vi "Photon-STR18_2_1.vi"() -> ()   [LabVIEW 2015]
uses:
  subVi/Menu.ctl
  <vilib>/Utility/file.llb/Write Delimited Spreadsheet (DBL).vi
panel:
  out "Size B":dbl
  out "Size A":dbl
  out "Duration A":dbl format="%.4f"
  out "Duration B":dbl format="%.4f"
  out "Total # of photons B":dbl
  out "Total # of photons A":dbl
  in  "Sample Time":i32=2
  out "b AxB":dbl format="%.4f"
  out "Correlacion 2":cluster{ext[], ext[]}(graph)
  out "< B >":dbl format="%.4f"
  out "< A >":dbl format="%.4f"
  out "Structura corregida":cluster{ext[], ext[]}(graph)
  in  "P":i32=64
  out "Numeric":i32
  out "sum A":dbl format="%#_10g"
  out "sum B":dbl format="%#_10g"
  out "Correlacion":cluster{ext[], ext[]}(graph)
  out "# of Channels":i32
  out "Duration":sgl
  in  "m":i32=2
  out "time":ext[](array[numeric])
  out "corr":ext[](array[numeric])
  out "d*(k)":dbl[][](array[numeric])
  out "Structura":cluster{ext[], ext[]}(graph)
  out "g(k) lineal":ext[](array[numeric])
  out "millisecond timer value":u32
  in  "EXIT":bool
  in  "Open File":bool
  in  "Analysis":u16(ring) items=["Auto correlation", "Cross correlation AxB"]
  out "elapsed time in min":dbl
  out "Elapsed time (s)":dbl
  # "PhotonSTR-18"
  # "Parameters"
  # "Output"
  # "Channel A"
  # "Channel B"
  # "V2.1"
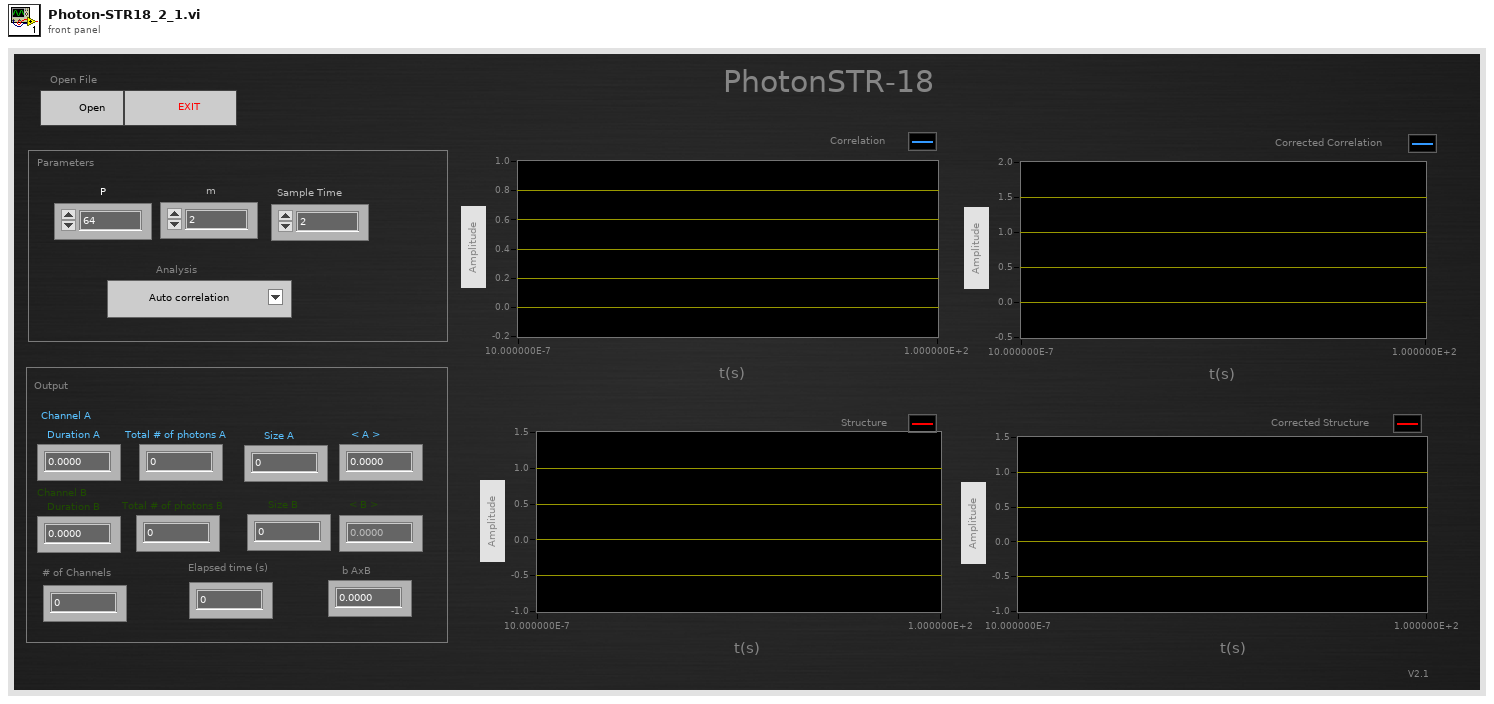
[diagram p1: front panel]
types:
  T1 = typedef "Menu.ctl" = enum16{"Init", "user action", "Load file", "Select range", "Process Photons(t)", "Process Segmentation", "Process Correlation ", "Save data", "Stop"}
  T2 = enum16{"open", "replace", "create", "open or create", "replace or create", "replace or create with confirmation"}
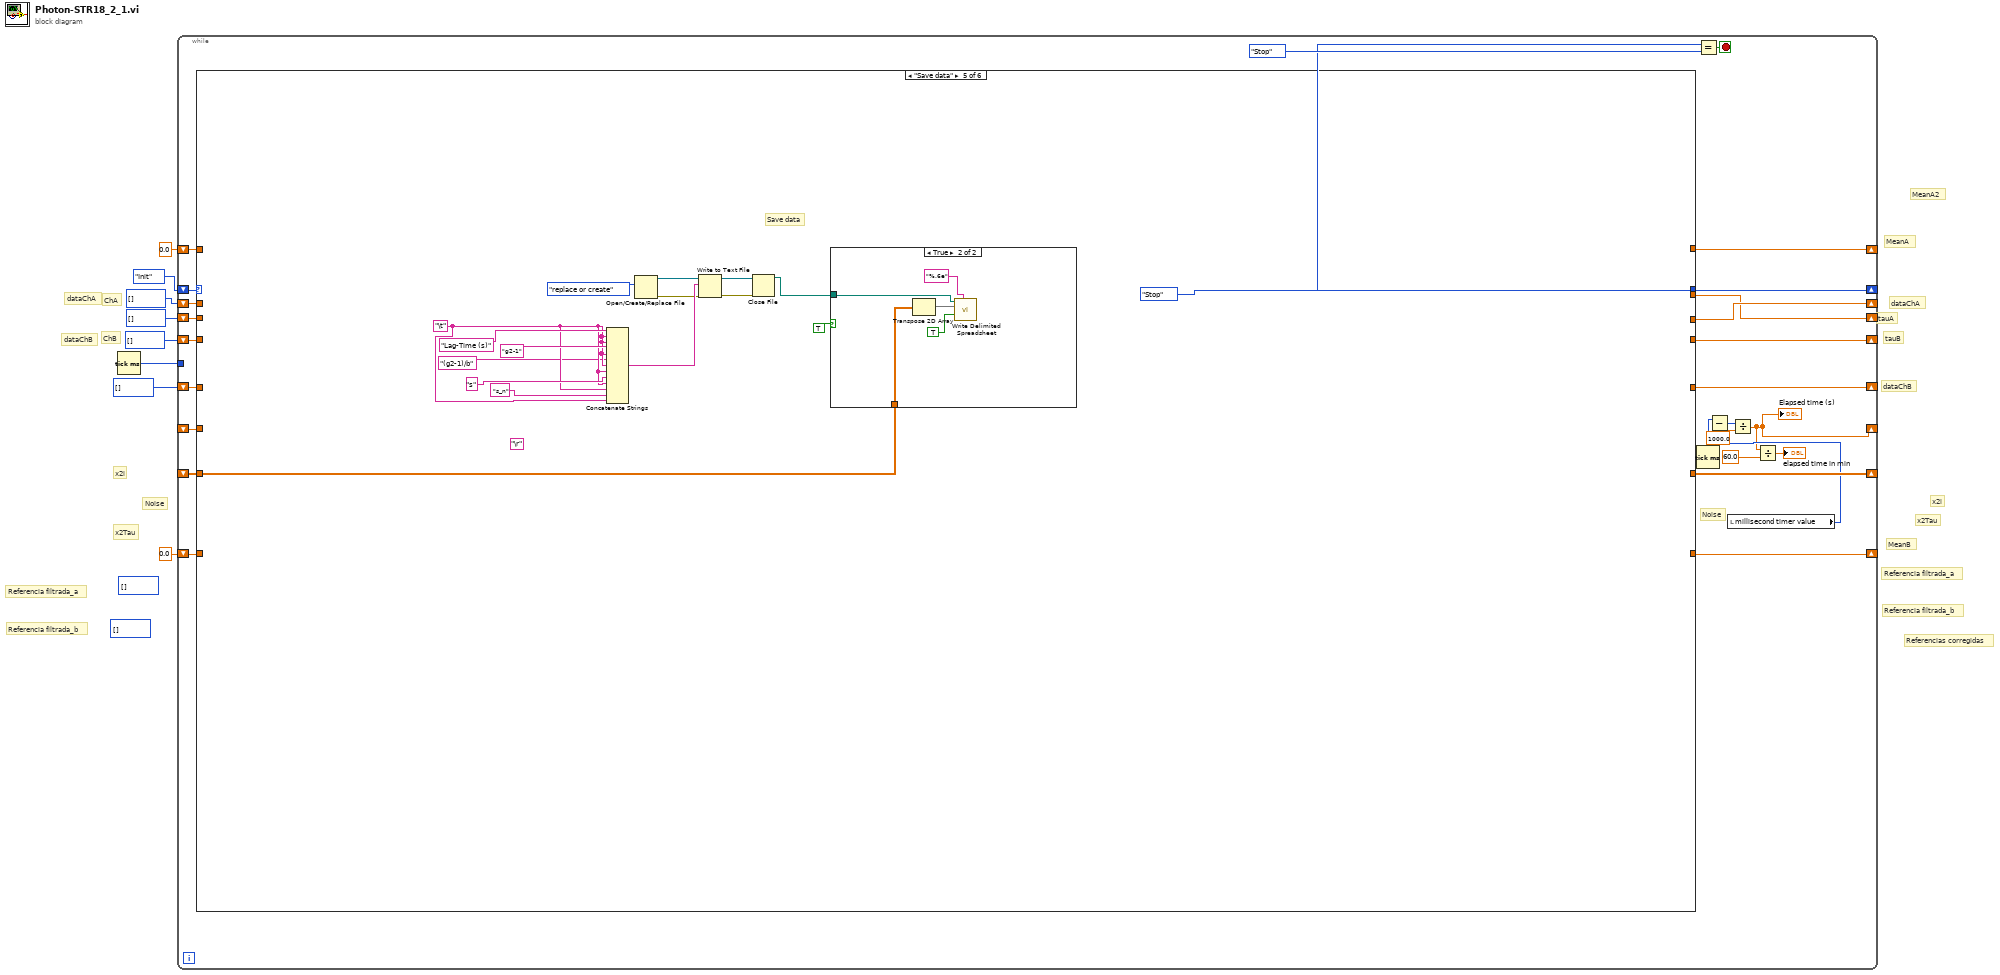
[diagram p0: block diagram]
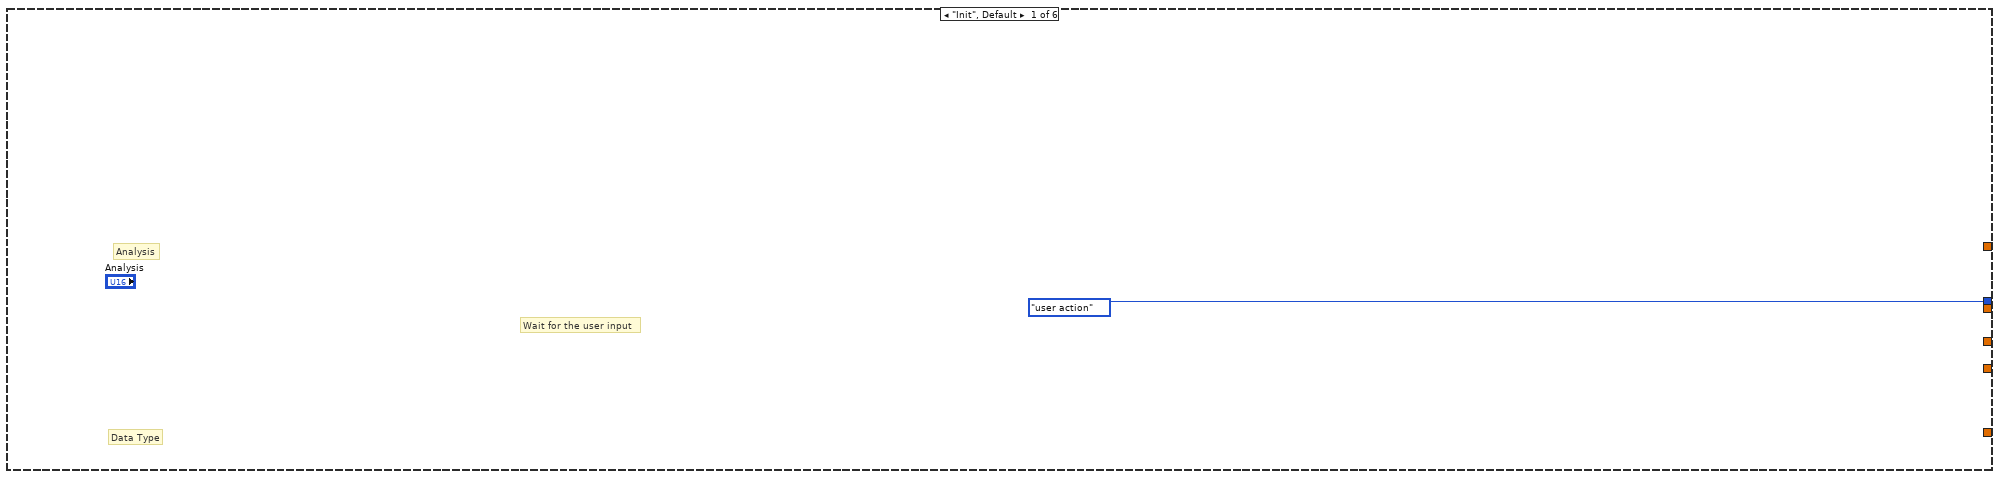
[diagram p2: hidden frame]
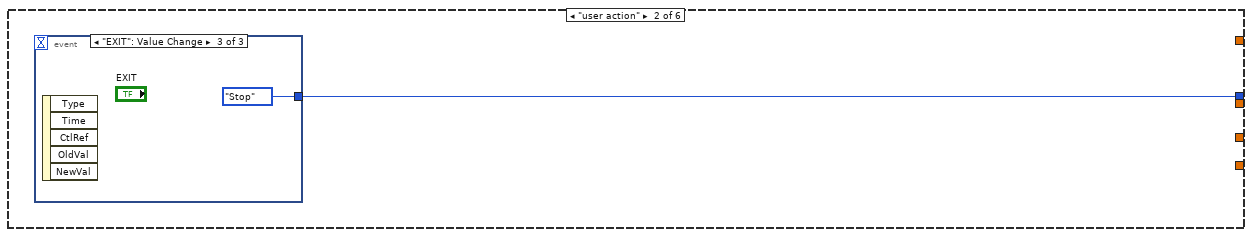
[diagram p3: hidden frame]
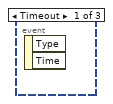
[diagram p4: hidden frame]
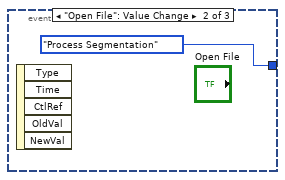
[diagram p5: hidden frame]
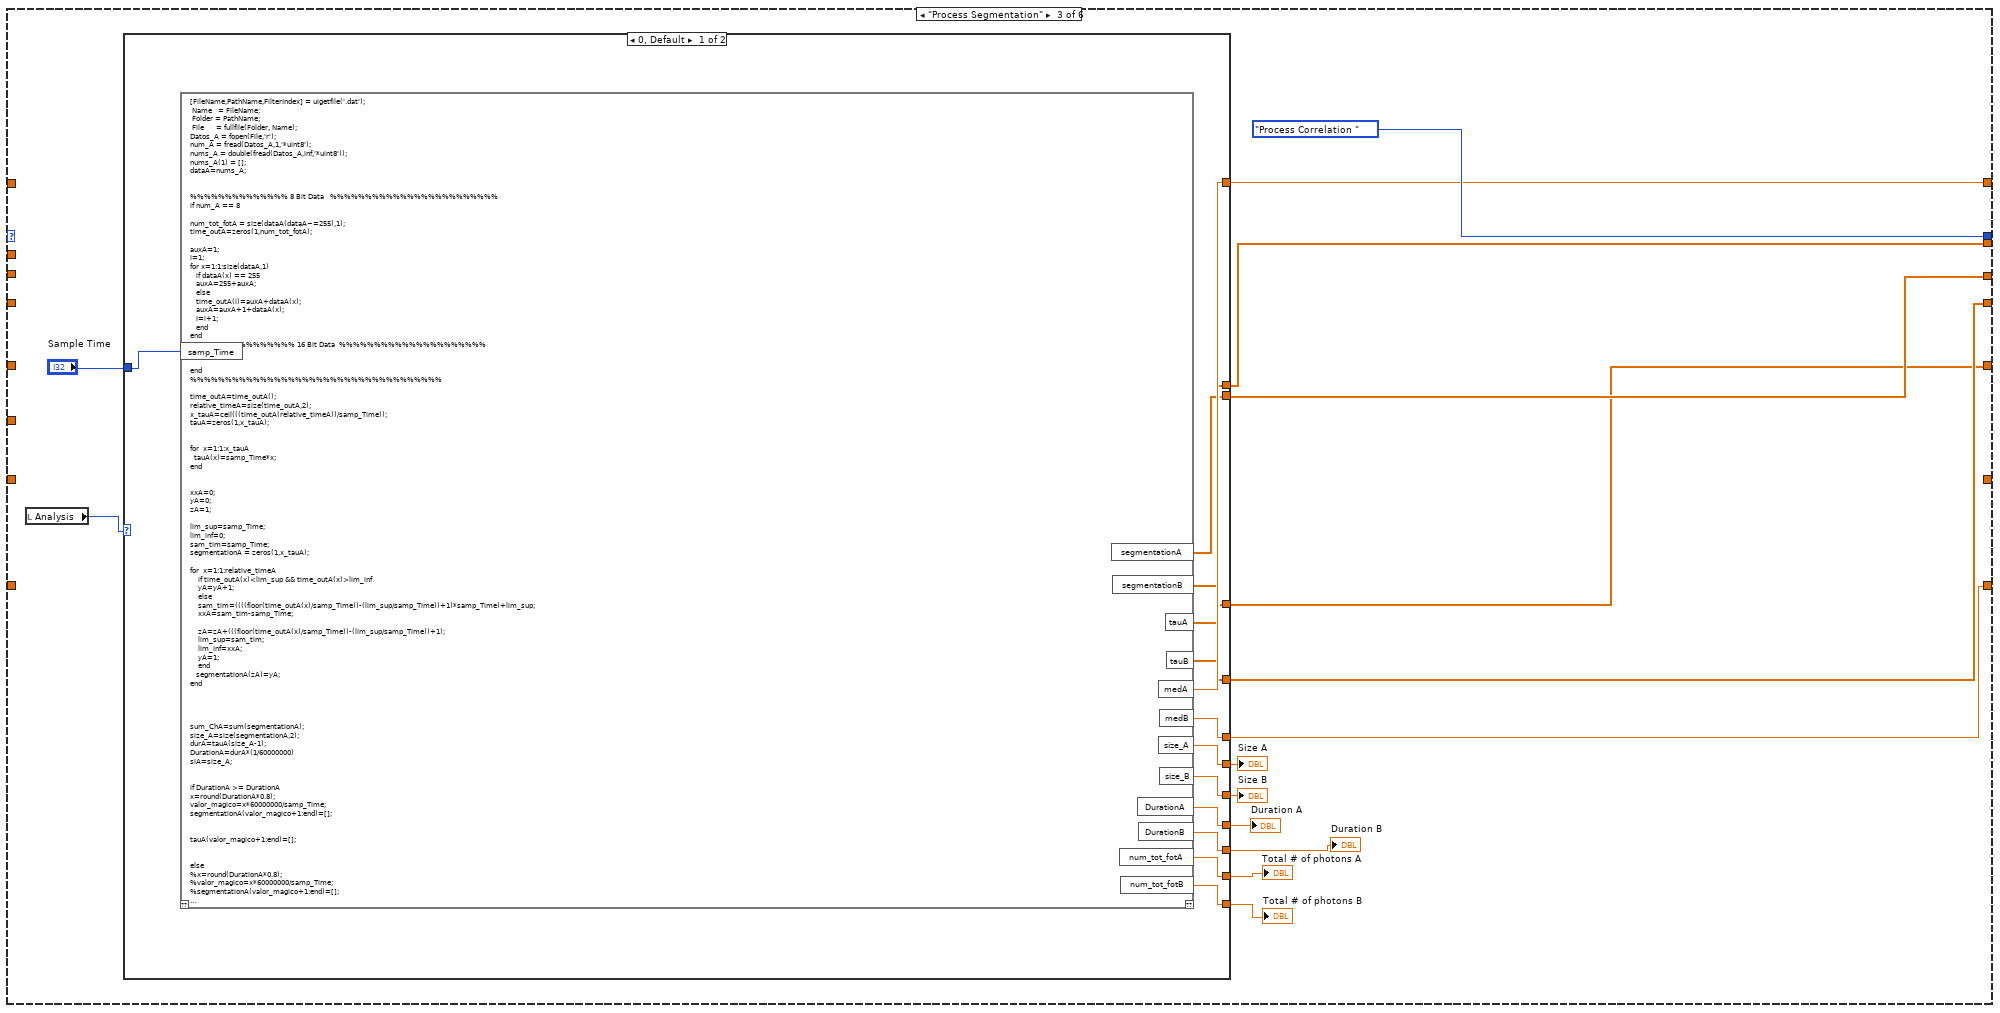
[diagram p6: hidden frame]
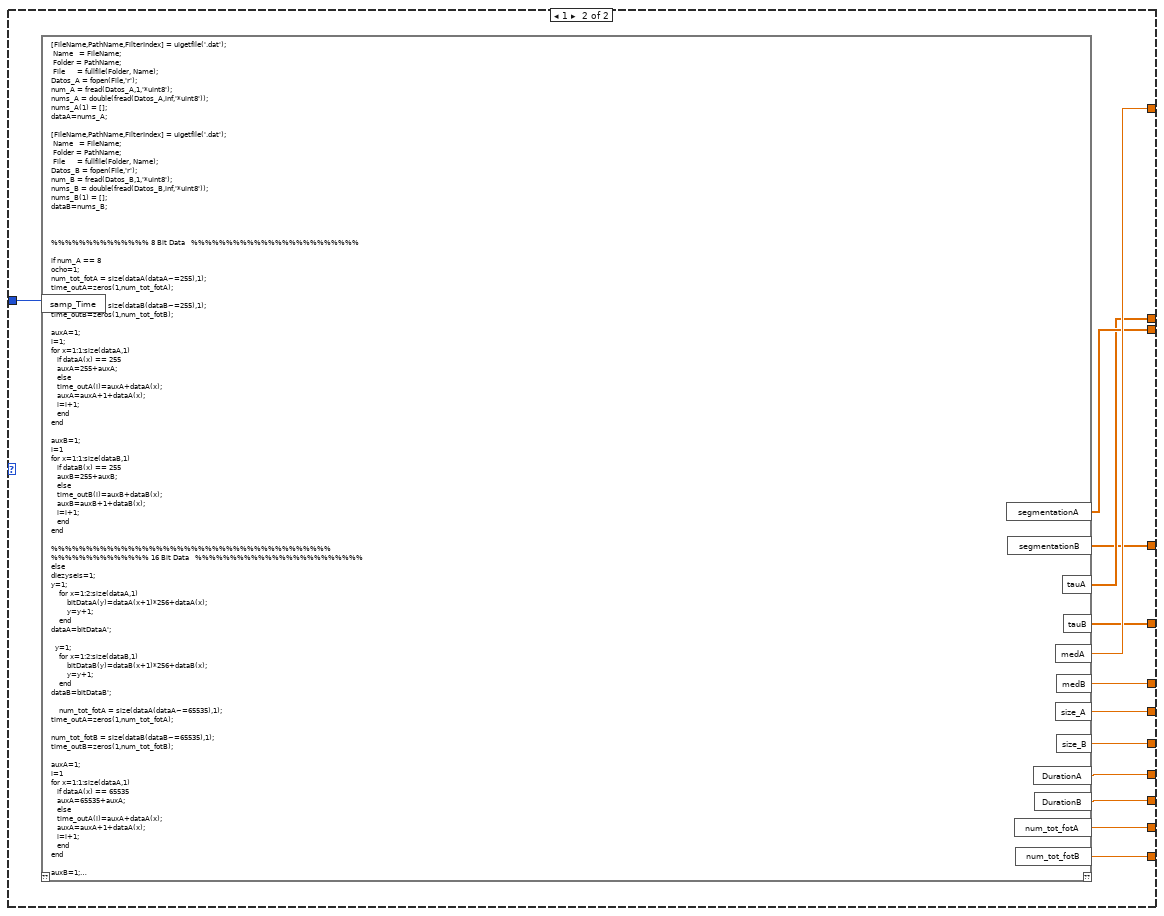
[diagram p7: hidden frame]
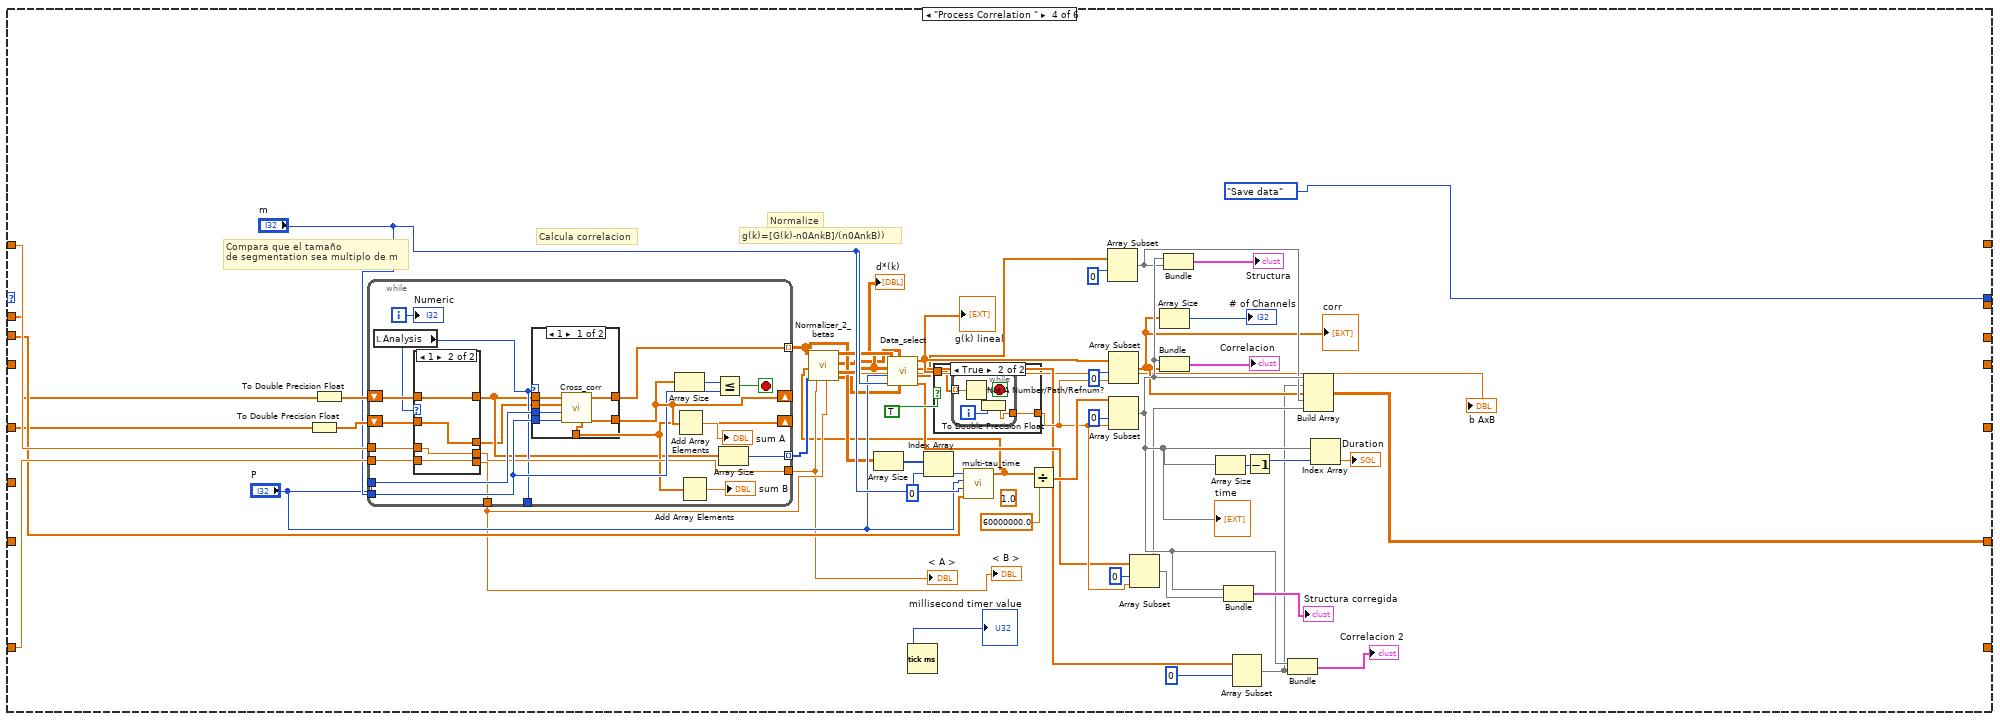
[diagram p8: hidden frame]
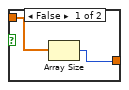
[diagram p9: hidden frame]
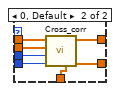
[diagram p10: hidden frame]
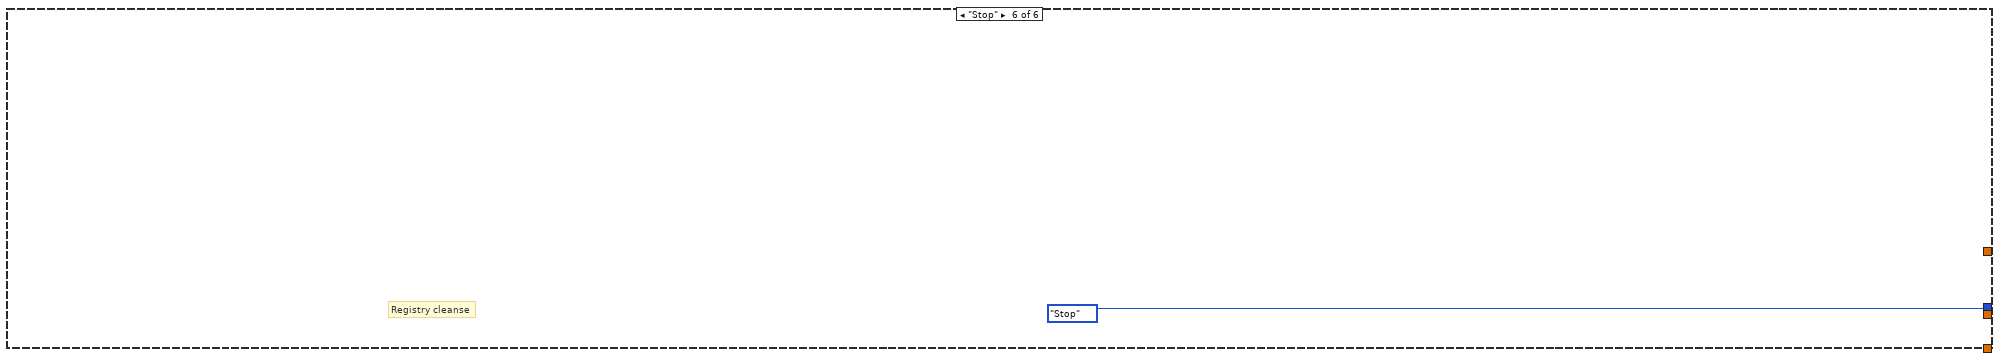
[diagram p13: hidden frame]
diagram:
  (unwired) u32[] [] ("Photon trace A")
  (unwired) u32[] [] ("Photon trace A")
  # "dataChB"
  # "dataChA"
  # "Referencias corregidas"
  # "Referencia filtrada_b"
  # "Referencia filtrada_a"
  # "Referencia filtrada_b"
  # "Referencia filtrada_a"
  # "Noise"
  # "x2Tau"
  # "x2i"
  # "x2Tau"
  # "x2i"
  # "MeanA2"
  # "MeanB"
  # "MeanA"
  # "tauB"
  # "tauA"
  # "ChB"
  # "dataChB"
  # "dataChA"
  # "ChA"
  n1 = Tick Count (ms)() -> (millisecond timer value=w5:u32)
  n2 = while {
    shift-right: [w32] -> _
    shift-left: Menu."Init" ("Menu") -> [w34]
    shift-right: [w30] -> _
    shift-left: u32[] [] ("Photon trace A") -> [w29]
    shift-right: [w28] -> _
    shift-left: u32[] [] ("Photon trace A") -> [w27]
    shift-right: [w16] -> _
    shift-left: _ -> [w26]
    tunnel: w5 -> [_]
    shift-right: [w20] -> _
    shift-left: u32[] [] ("Photon trace A") -> [w19]
    shift-right: [w18] -> _
    shift-left: u32[] [] ("Photon trace A") -> [w17]
    shift-right: [w13] -> _
    shift-left: _ -> [w15]
    shift-right: [w12] -> _
    shift-left: 0.0 ("mean") -> [w10]
    shift-right: [w11] -> _
    shift-left: 0.0 ("mean") -> [w9]
    stop <- w31 stop-if-true
    # "Noise"
    n3 = case shown="\"Save data\"" w34 {
      tunnel: [Menu."user action" ("Menu") w36 Menu."Process Correlation " ("Menu") Menu."Save data" ("Menu") Menu."Stop" ("Menu") Menu."Stop" ("Menu")] -> w32
      tunnel: [_ _ w42 _ _ _] -> w30
      tunnel: w29 -> [_ _ _ w83 _ _]
      tunnel: [_ _ w39 _ _ _] -> w28
      tunnel: w27 -> [_ _ _ w109 _ _]
      tunnel: [_ _ _ w129 _ _] -> w16
      tunnel: w26 -> [_ _ _ _ w195 _]
      tunnel: [_ _ w41 _ _ _] -> w20
      tunnel: w19 -> [_ _ _ _ _ _]
      tunnel: [_ _ w40 _ _ _] -> w18
      tunnel: w17 -> [_ _ _ w105 _ _]
      tunnel: w15 -> [_ _ _ _ _ _]
      tunnel: [_ _ w51 _ _ _] -> w12
      tunnel: [_ _ w50 _ _ _] -> w11
      tunnel: w10 -> [_ _ _ w128 _ _]
      tunnel: w9 -> [_ _ _ w127 _ _]
      frame "Init", Default {
        # "Data Type"
        # "Analysis"
        # "Wait for the user input"
      }
      frame "user action" {
        n4 = event shown="[2] \"EXIT\": Value Change" {
          selector: _ -> [_ _ _]
          dyn-events: _ -> [_ _ _]
          timeout: _ -> [_ _ _]
          tunnel: [_ Menu."Process Segmentation" ("Menu") Menu."Stop" ("Menu")] -> w36
          event Timeout {
            n5 = event-data() -> ()  [unwired: 1 in, 2 out]
          }
          event "Open File": Value Change {
            n6 = event-data() -> ()  [unwired: 1 in, 5 out]
          }
          event "EXIT": Value Change {
            n7 = event-data() -> ()  [unwired: 1 in, 5 out]
          }
        }
      }
      frame "Process Segmentation" {
        n8 = local read "Analysis"() -> (w43:u16)
        n9 = case shown="0, Default" w43 {
          tunnel: "Sample Time" -> [w66 w79]
          tunnel: [w58 w78] -> w51
          tunnel: [w59 w77] -> w50
          tunnel: [w64 w76] -> w49
          tunnel: [w65 w75] -> w48
          tunnel: [w61 w74] -> w47
          tunnel: [w60 w73] -> w46
          tunnel: [w56 w72] -> w42
          tunnel: [w57 w71] -> w39
          tunnel: [w54 w70] -> w41
          tunnel: [w55 w69] -> w40
          tunnel: [w62 w68] -> w45
          tunnel: [w63 w67] -> w44
          frame 0, Default {
            n10 = script code="[FileName,PathName,FilterIndex] = uigetfile('.dat');\n Name   = FileName;\n Folder = PathName;\n File      = fullfile(Folder, Name);         \nDatos_A = fopen(File,'r');  \nnum_A = fread(Datos_A,1,'*uint8');\nnums_A = double(fread(Datos_A,inf,'*uint8'));\nnums_A(1) = []; \ndataA=nums_A;\n\n\n%%%%%%%%%%%%%% 8 Bit Data   %%%%%%%%%%%%%%%%%%%%%%%%\nif num_A == 8 \n\nnum_tot_fotA = size(dataA(dataA~=255),1); \ntime_outA=zeros(1,num_tot_fotA);\n\nauxA=1;\ni=1;\nfor x=1:1:size(dataA,1)\n   if dataA(x) == 255\n   auxA=255+auxA;    \n   else\n   time_outA(i)=auxA+dataA(x);\n   auxA=auxA+1+dataA(x);   \n   i=i+1;\n   end\nend\n%%%%%%%%%%%%%%% 16 Bit Data  %%%%%%%%%%%%%%%%%%%%%\n\n\nend\n%%%%%%%%%%%%%%%%%%%%%%%%%%%%%%%%%%%%\n\ntime_outA=time_outA();\nrelative_timeA=size(time_outA,2);\nx_tauA=ceil(((time_outA(relative_timeA))/samp_Time));\ntauA=zeros(1,x_tauA);\n\n\nfor  x=1:1:x_tauA\n  tauA(x)=samp_Time*x;   \nend\n\n\nxxA=0;\nyA=0;\nzA=1;\n\nlim_sup=samp_Time;\nlim_inf=0;\nsam_tim=samp_Time;\nsegmentationA = zeros(1,x_tauA);\n\nfor  x=1:1:relative_timeA\n    if time_outA(x)<lim_sup && time_outA(x)>lim_inf\n    yA=yA+1;    \n    else\n    sam_tim=((((floor(time_outA(x)/samp_Time))-(lim_sup/samp_Time))+1)*samp_Time)+lim_sup;\n    xxA=sam_tim-samp_Time;\n    \n    zA=zA+(((floor(time_outA(x)/samp_Time))-(lim_sup/samp_Time))+1);\n    lim_sup=sam_tim;\n    lim_inf=xxA;    \n    yA=1;\n    end    \n   segmentationA(zA)=yA;\nend \n                          \n\n\n\nsum_ChA=sum(segmentationA);\nsize_A=size(segmentationA,2);\ndurA=tauA(size_A-1);\nDurationA=durA*(1/60000000)\nsiA=size_A;\n\n\nif DurationA >= DurationA\nx=round(DurationA*0.8);\nvalor_magico=x*60000000/samp_Time; \nsegmentationA(valor_magico+1:end)=[];\n\n\ntauA(valor_magico+1:end)=[];\n\n\nelse\n%x=round(DurationA*0.8);\n%valor_magico=x*60000000/samp_Time; \n%segmentationA(valor_magico+1:end)=[];\n\n\n%tauA(valor_magico+1:end)=[];\n\nend\n\nmedA=mean(segmentationA);\nmedB=medA;\n\nsegmentationB=segmentationA;\ntauB=tauA;\nsize_B=size_A;\nDurationB=DurationA;\nnum_tot_fotB = num_tot_fotA ;"("samp_Time"=w66) -> ("segmentationA"=w56:dbl[], "segmentationB"=w55:dbl[], "tauA"=w57:dbl[], "tauB"=w54:dbl[], "medA"=w58:dbl, "medB"=w59:dbl, "DurationA"=w62:dbl, "DurationB"=w63:dbl, "num_tot_fotA"=w64:dbl, "num_tot_fotB"=w65:dbl, "size_A"=w60:dbl, "size_B"=w61:dbl)  [unwired: 1 in, 1 out]
          }
          frame 1 {
            n11 = script code="[FileName,PathName,FilterIndex] = uigetfile('.dat');\n Name   = FileName;\n Folder = PathName;\n File      = fullfile(Folder, Name);         \nDatos_A = fopen(File,'r');  \nnum_A = fread(Datos_A,1,'*uint8');\nnums_A = double(fread(Datos_A,inf,'*uint8'));\nnums_A(1) = []; \ndataA=nums_A;\n\n[FileName,PathName,FilterIndex] = uigetfile('.dat');\n Name   = FileName;\n Folder = PathName;\n File      = fullfile(Folder, Name);         \nDatos_B = fopen(File,'r');  \nnum_B = fread(Datos_B,1,'*uint8');\nnums_B = double(fread(Datos_B,inf,'*uint8'));\nnums_B(1) = []; \ndataB=nums_B;\n\n\n\n%%%%%%%%%%%%%% 8 Bit Data   %%%%%%%%%%%%%%%%%%%%%%%%\n\nif num_A == 8 \nocho=1;\nnum_tot_fotA = size(dataA(dataA~=255),1); \ntime_outA=zeros(1,num_tot_fotA);\n\nnum_tot_fotB = size(dataB(dataB~=255),1); \ntime_outB=zeros(1,num_tot_fotB);\n\nauxA=1;\ni=1;\nfor x=1:1:size(dataA,1)\n   if dataA(x) == 255\n   auxA=255+auxA;    \n   else\n   time_outA(i)=auxA+dataA(x);\n   auxA=auxA+1+dataA(x);   \n   i=i+1;\n   end\nend\n\nauxB=1;\ni=1\nfor x=1:1:size(dataB,1)\n   if dataB(x) == 255\n   auxB=255+auxB;    \n   else\n   time_outB(i)=auxB+dataB(x);\n   auxB=auxB+1+dataB(x);   \n   i=i+1;\n   end\nend\n\n%%%%%%%%%%%%%%%%%%%%%%%%%%%%%%%%%%%%%%%%\n%%%%%%%%%%%%%% 16 Bit Data   %%%%%%%%%%%%%%%%%%%%%%%%\nelse\ndiezyseis=1;\ny=1;\n    for x=1:2:size(dataA,1)\n        bitDataA(y)=dataA(x+1)*256+dataA(x);\n        y=y+1;\n    end\ndataA=bitDataA';\n\n  y=1;\n    for x=1:2:size(dataB,1)\n        bitDataB(y)=dataB(x+1)*256+dataB(x);\n        y=y+1;\n    end\ndataB=bitDataB';\n\n    num_tot_fotA = size(dataA(dataA~=65535),1); \ntime_outA=zeros(1,num_tot_fotA);\n\nnum_tot_fotB = size(dataB(dataB~=65535),1); \ntime_outB=zeros(1,num_tot_fotB);\n\nauxA=1;\ni=1\nfor x=1:1:size(dataA,1)\n   if dataA(x) == 65535\n   auxA=65535+auxA;    \n   else\n   time_outA(i)=auxA+dataA(x);\n   auxA=auxA+1+dataA(x);   \n   i=i+1;\n   end\nend\n\nauxB=1;\ni=1\nfor x=1:1:size(dataB,1)\n   if dataB(x) == 65535\n   auxB=65535+auxB;    \n   else\n   time_outB(i)=auxB+dataB(x);\n   auxB=auxB+1+dataB(x);   \n   i=i+1;\n   end\nend\n\nend \n%%%%%%%%%%%%%% 16 Bit Data   %%%%%%%%%%%%%%%%%%%%%%%%\n\n\ntime_outA=time_outA();\nrelative_timeA=size(time_outA,2);\nx_tauA=ceil(((time_outA(relative_timeA))/samp_Time));\ntauA=zeros(1,x_tauA);\n\ntime_outB=time_outB();\nrelative_timeB=size(time_outB,2);\nx_tauB=ceil(((time_outB(relative_timeB))/samp_Time));\ntauB=zeros(1,x_tauB);\n\nfor  x=1:1:x_tauA\n  tauA(x)=samp_Time*x;   \nend\n\nfor  x=1:1:x_tauB\n  tauB(x)=samp_Time*x;   \nend\n\n\nxxA=0;\nyA=0;\nzA=1;\n\nxxB=0;\nyB=0;\nzB=1;\n\nlim_sup=samp_Time;\nlim_inf=0;\nsam_tim=samp_Time;\nsegmentationA = zeros(1,x_tauA);\n\nfor  x=1:1:relative_timeA\n    if time_outA(x)<lim_sup && time_outA(x)>lim_inf\n    yA=yA+1;    \n    else\n    sam_tim=((((floor(time_outA(x)/samp_Time))-(lim_sup/samp_Time))+1)*samp_Time)+lim_sup;\n    xxA=sam_tim-samp_Time;\n    \n    zA=zA+(((floor(time_outA(x)/samp_Time))-(lim_sup/samp_Time))+1);\n    lim_sup=sam_tim;\n    lim_inf=xxA;    \n    yA=1;\n    end    \n   segmentationA(zA)=yA;\nend \n                          \nlim_sup=samp_Time;\nlim_inf=0;\nsam_tim=samp_Time;\nsegmentationB = zeros(1,x_tauB);\n\nfor  x=1:1:relative_timeB\n    if time_outB(x)<lim_sup && time_outB(x)>lim_inf\n    yB=yB+1;    \n    else\n    sam_tim=((((floor(time_outB(x)/samp_Time))-(lim_sup/samp_Time))+1)*samp_Time)+lim_sup;\n    xxB=sam_tim-samp_Time;\n    \n    zB=zB+(((floor(time_outB(x)/samp_Time))-(lim_sup/samp_Time))+1);\n    lim_sup=sam_tim;\n    lim_inf=xxB;    \n    yB=1;\n    end    \n   segmentationB(zB)=yB;\nend \n\nsum_ChA=sum(segmentationA);\nsize_A=size(segmentationA,2);\ndurA=tauA(size_A-1);\nDurationA=durA*(1/60000000)\nsiA=size_A;\n\nsum_ChB=sum(segmentationB);\nsize_B=size(segmentationB,2);\ndurB=tauB(size_B-1);\nDurationB=durB*(1/60000000)\nsiB=size_B;\n\nif DurationA >= DurationB\nx=round(DurationB*0.8);\nvalor_magico=x*60000000/samp_Time; \nsegmentationA(valor_magico+1:end)=[];\nsegmentationB(valor_magico+1:end)=[];\n\ntauA(valor_magico+1:end)=[];\ntauB(valor_magico+1:end)=[];\n\nelse\nx=round(DurationA*0.8);\nvalor_magico=x*60000000/samp_Time; \nsegmentationA(valor_magico+1:end)=[];\nsegmentationB(valor_magico+1:end)=[];\n\ntauA(valor_magico+1:end)=[];\ntauB(valor_magico+1:end)=[];\n\nend\n\nmedA=mean(segmentationA);\nmedB=mean(segmentationB);"("samp_Time"=w79) -> ("segmentationA"=w72:dbl[], "segmentationB"=w69:dbl[], "tauA"=w71:dbl[], "tauB"=w70:dbl[], "medA"=w78:dbl, "medB"=w77:dbl, "DurationA"=w68:dbl, "DurationB"=w67:dbl, "num_tot_fotA"=w76:dbl, "num_tot_fotB"=w75:dbl, "size_A"=w73:dbl, "size_B"=w74:dbl)  [unwired: 1 in, 1 out]
          }
        }
        "Total # of photons A" <- w49
        "Total # of photons B" <- w48
        "Duration B" <- w44
        "Duration A" <- w45
        "Size A" <- w46
        "Size B" <- w47
      }
      frame "Process Correlation " {
        (unwired) 1.0 ("y")
        # "Calcula correlacion"
        # "g(k)=[G(k)-n0AnkB]/(n0AnkB))"
        # "Normalize"
        # "Compara que el tamaño\nde segmentation sea multiplo de m"
        n12 = To Double Precision Float(number=w105) -> (double precision float=w116:dbl[])
        n13 = To Double Precision Float(number=w83) -> (double precision float=w117:dbl[])
        n14 = while {
          tunnel: [w157] -> w101 mode=indexing
          shift-right: [w153] -> _
          shift-left: w117 -> [w150]
          tunnel: "m" -> [w147]
          tunnel: "P" -> [w148]
          tunnel: [w155] -> w106 mode=indexing
          shift-right: [w142] -> _
          shift-left: w116 -> [w149]
          tunnel: w128 -> [w146]
          tunnel: w127 -> [w145]
          tunnel: [w144] -> w82
          tunnel: [w143] -> w94
          tunnel: [w141] -> _
          i -> [w154]
          stop <- w158 stop-if-true
          n15 = local read "Analysis"() -> (w141:u16)
          n16 = case shown="1" w141 {
            tunnel: w150 -> [w176 w180]
            tunnel: [w176 w180] -> w140
            tunnel: [w175 w179] -> w139
            tunnel: w149 -> [w175 w179]
            tunnel: w146 -> [w174 w178]
            tunnel: w145 -> [w173 w177]
            tunnel: [w174 w178] -> w144
            tunnel: [w173 w177] -> w143
            frame 0, Default {
            }
            frame 1 {
            }
          }
          n17 = case shown="1" w141 {
            tunnel: [w165 w172] -> w157
            tunnel: w148 -> [w160 w167]
            tunnel: w147 -> [w159 w166]
            tunnel: [w164 w171] -> w153
            tunnel: [w163 w170] -> w142
            tunnel: w139 -> [w161 w168]
            tunnel: w140 -> [w162 w169]
            frame 1 {
              n18 = call "Cross_corr.vi"("m"=w159, "P"=w160, "input B"=w161, "input A"=w162) -> ("Sn A"=w164:dbl[], "Acc"=w165:dbl[], "Sn B"=w163:dbl[])  [unwired: 5 in]
            }
            frame 0, Default {
              n19 = call "Cross_corr.vi"("m"=w166, "P"=w167, "input B"=w168, "input A"=w169) -> ("Sn A"=w171:dbl[], "Acc"=w172:dbl[], "Sn B"=w170:dbl[])  [unwired: 5 in]
            }
          }
          n20 = Array Size(array=w153) -> (size(s)=w156:i32)
          n21 = Add Array Elements(numeric array=w153) -> (sum=→"sum A":dbl)
          n22 = Add Array Elements(numeric array=w142) -> (sum=→"sum B":dbl)
          n23 = Less Or Equal?(x=w156, y=w147) -> (x <= y?=w158:bool)
          n24 = Array Size(array=w140) -> (size(s)=w155:i32)
          "Numeric" <- w154
        }
        "< A >" <- w82
        "< B >" <- w94
        n25 = Array Size(array=w101) -> (size(s)=w102:i32[])
        n26 = Tick Count (ms)() -> (millisecond timer value=→"millisecond timer value":u32)
        n27 = Index Array(array=w102, index=0) -> (element=w118:i32)
        n28 = call "multi-tau_time.vi"("tau"=w109, "m"="m", "P"="P", "No. of shift registers"=w118) -> ("time multi-tau"=w80:ext[])  [unwired: 7 in]
        n29 = call "Normalizer_2_betas.vi"("Acc"=w101, "Time"=w80, "Tamaño Sn"=w106, "AvgA"=w82, "AvgB"=w94) -> ("bA_B"=→"b AxB":dbl, "g(k)_2"=w104:dbl[][], "s(k)_n"=w95:dbl[][], "s(k)"=w103:dbl[][], "g(k)"=w93:dbl[][])  [unwired: 10 in]
        "d*(k)" <- w103
        n30 = call "Data_select.vi"("g(k) in 2"=w93, "s(k) Corregido"=w95, "m"="m", "P"="P", "s(k) in"=w103, "g(k) in"=w104) -> ("s(k) lineal Corregido"=w97:ext[], "s(k) lineal"=w81:ext[], "g(k)lineal_2"=w91:ext[], "g(k) lineal"=w110:ext[])  [unwired: 2 in]
        "g(k) lineal" <- w110
        n31 = case shown="True" TRUE {
          tunnel: w110 -> [w132 w134]
          tunnel: [w131 w133] -> w98
          frame False {
            n32 = Array Size(array=w132) -> (size(s)=w131:i32)
          }
          frame True {
            n33 = while {
              tunnel: w134 -> [w138] mode=indexing
              tunnel: [w135] -> w133
              i -> [w136]
              stop <- w137 stop-if-true
              n34 = Not A Number/Path/Refnum?(number/path/refnum=w138) -> (NaN/Path/Refnum?=w137:bool)
              n35 = To Double Precision Float(number=w136) -> (double precision float=w135:dbl)
            }
          }
        }
        n36 = Divide(x=w80, y=60000000.0) -> (x/y=w100:ext[])
        n37 = Array Subset(array=w81, index=0) -> (w87:ext[])  [unwired: 1 in]
        n38 = Array Subset(array=w110, index=0, length=w98) -> (w86:ext[])
        "corr" <- w86
        n39 = Array Subset(array=w100, index=0, length=w98) -> (w90:ext[])
        "time" <- w90
        n40 = Array Subset(array=w97, index=0, length=w98) -> (w88:ext[])
        n41 = Array Size(array=w86) -> (size(s)=→"# of Channels":i32)
        n42 = Bundle(w90, w86) -> (→"Correlacion":cluster{ext[], ext[]})  [unwired: 1 in]
        n43 = Bundle(w90, w87) -> (→"Structura":cluster{ext[], ext[]})  [unwired: 1 in]
        n44 = Array Size(array=w90) -> (size(s)=w124:i32)
        n45 = Bundle(w90, w88) -> (→"Structura corregida":cluster{ext[], ext[]})  [unwired: 1 in]
        n46 = Array Subset(array=w91, index=0) -> (w85:ext[])  [unwired: 1 in]
        n47 = Decrement(x=w124) -> (x-1=w123:i32)
        n48 = Bundle(w90, w85) -> (→"Correlacion 2":cluster{ext[], ext[]})  [unwired: 1 in]
        n49 = Build Array(w90, w85, w86, w87, w88) -> (w129:ext[][])
        n50 = Index Array(array=w90, index=w123) -> (element=→"Duration":ext)
      }
      frame "Save data" {
        w182 = "\t"
        (unwired) "\r"
        # "Save data"
        n51 = Concatenate Strings("Lag-Time (s)" ("string"), w182, w182, "g2-1" ("string"), w182, "(g2-1)/b" ("string"), w182, w182, "s" ("string"), w182, w182, "s_n" ("string"), w182) -> (w194:string)
        n52 = Open/Create/Replace File(operation (0:open)=T2."replace or create") -> (refnum out=w193:refnum<file>, error out=w192:errorcluster)  [unwired: 5 in, 1 out]
        n53 = Write to Text File(file (use dialog)=w193, text=w194, error in=w192) -> (refnum out=w191:refnum<file>, error out=w190:errorcluster)  [unwired: 1 in, 1 out]
        n54 = Close File(refnum=w191, error in=w190) -> (path=w189:path)  [unwired: 1 out]
        n55 = case shown="True" TRUE {
          tunnel: w195 -> [_ w201]
          tunnel: w189 -> [_ w197]
          frame False {
          }
          frame True {
            n56 = Transpose 2D Array(2D array=w201) -> (transposed array=w200:ext[][])
            n57 = call-poly <vilib>:"Write Delimited Spreadsheet.vi"("file path (dialog if empty)"=w197, "format (%.3f)"="%.6e", "2D data"=w200, "append to file? (F)"=TRUE) -> ()  [unwired: 10 in, 2 out]
          }
        }
      }
      frame "Stop" {
        # "Registry cleanse"
      }
    }
    n58 = Tick Count (ms)() -> (millisecond timer value=w23:u32)
    n59 = Equal?(x=w32, y=Menu."Stop" ("Menu")) -> (x = y?=w31:bool)
    n60 = local read "millisecond timer value"() -> (w14:u32)
    n61 = Subtract(x=w23, y=w14) -> (x-y=w25:u32)
    n62 = Divide(x=w25, y=1000.0) -> (x/y=w13:dbl)
    "Elapsed time (s)" <- w13
    n63 = Divide(x=w13, y=60.0) -> (x/y=→"elapsed time in min":dbl)
  }
